vi "NI VeriStand - Open Error Message Notification.vi"(8 "error in (no error)":errorcluster, 11 "MacroPlayer in":T2) -> (0 "error out":errorcluster, 2 "ErrorMessage Refs":T1, 3 "MacroPlayer out":T2)   [LabVIEW 2020, in "NI_VS MacroPlayerAPI.lvlib"]
doc: "Opens a reference to error messages the Macro Player sends. This VI returns a user event that you can register and wire to an Event structure."
uses:
  <vilib>/NI VeriStand/Execution/MacroPlayer/NI_VS MacroPlayerAPI.lvlib
  <vilib>/NI VeriStand/Execution/MacroPlayer/MacroPlayerAPI.ctl
  NationalInstruments.VeriStand.ClientAPI
  <vilib>/NI VeriStand/Execution/MacroPlayer/ErrorMessage Refs.ctl
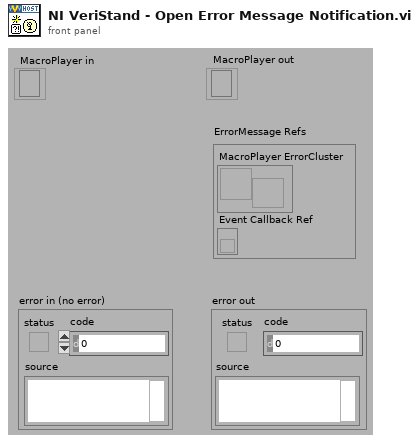
[diagram p1: front panel]
types:
  T1 = typedef "NI_VS MacroPlayerAPI.lvlib/ErrorMessage Refs.ctl" = cluster{"MacroPlayer ErrorCluster":refnum<user-event>, "Event Callback Ref":refnum<k27>}
  T2 = typedef "NI_VS MacroPlayerAPI.lvlib/MacroPlayerAPI.ctl" = refnum<k24>
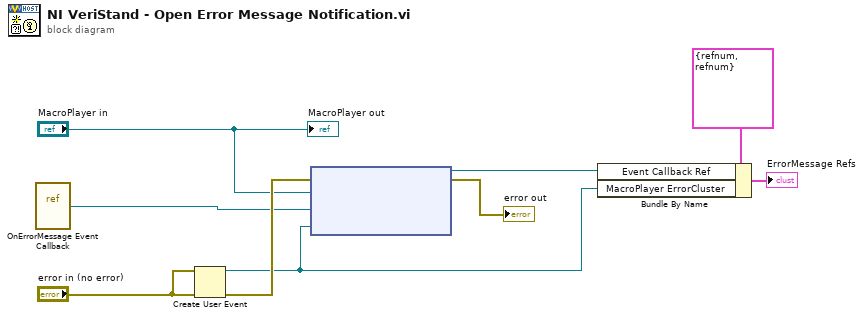
[diagram p0: block diagram]
diagram:
  n1 = vi-ref <vilib>:"OnErrorMessage Event Callback.vi"() -> ("vi reference"=w5:refnum<vi>)
  n2 = Create User Event(user event datatype="error in (no error)", error in="error in (no error)") -> (user event=w3:refnum<user-event>, error out=w9:errorcluster)
  n3 = node(w9, "MacroPlayer in", w5, w3) -> (w4:refnum<k27>, →"error out":errorcluster)  [unwired: 1 in]
  n4 = Bundle By Name(cluster=T1 {"MacroPlayer ErrorCluster"=refnum, "Event Callback Ref"=refnum} ("ErrorMessage Refs"), "Event Callback Ref"=w4, "MacroPlayer ErrorCluster"=w3) -> (→"ErrorMessage Refs":T1)
  "MacroPlayer out" <- "MacroPlayer in"
